vi "Periodic Tasks.vi"(8 "error in":errorcluster) -> ()   [LabVIEW 2016]
doc: "This VI runs in parallel to other tasks. It can contain as many user-defined periodic loops as you need. These can carry out PID or other sorts of timed response."
uses:
  <vilib>/Rock Robotics/WPI/AnalogOutput/WPI_AnalogOutputChannel.ctl
  <vilib>/Platform/TimedLoop/XDataNode/timing_clust.ctl
  <vilib>/Platform/TimedLoop/XDataNode/nitl_modes.ctl
  <vilib>/Platform/TimedLoop/XDataNode/wakeup.ctl
  <vilib>/Waveform/WDTFileIO.llb/Read Waveform from File.vi
  Robot Global Data.vi
  <vilib>/platform/TimedLoop/XDataNode/XDataNode.xnode
  <vilib>/Platform/TimedLoop/XDataNode/XDNodeRunTimeDep.lvlib
panel:
  in  "Volume":dbl(slide)=3.5 scale=0.0..3.0
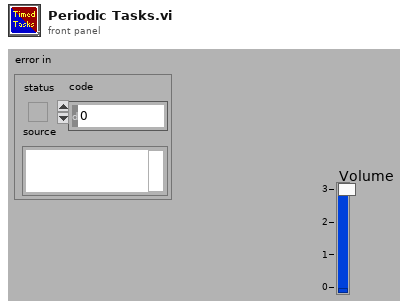
[diagram p1: front panel]
types:
  T1 = typedef "WPI_AnalogOutputChannel.ctl" = enum8{"AO MXP 0", "AO MXP 1", "Invalid"}
  T2 = typedef "JoystickData.ctl" = cluster{"X":dbl, "Y":dbl, "Z":dbl, "RestartMusic":bool}
  T3 = typedef "XDNodeRunTimeDep.lvlib/timing_clust.ctl" = cluster{"Expected End [f-1]":u64, "Actual End [f-1]":u64, "Finished Late? [f-1]":bool, "Expected End [i-1]":u64, "Actual End [i-1]":u64, "Finished Late? [i-1]":bool, "Expected Start [i]":u64, "Actual Start [i]":u64, "Expected Start [f]":u64, "Actual Start [f]":u64, "Source Name":string, "Structure Name":string, "Period":i64, "Deadline":i64, "Offset":i64, "Start":i64, "Priority":i32, "Timeout":i32, "Mode":T4, "Wakeup Reason":T5, "Error":errorcluster, "Source Type":string, "Secondary Source Type":string, "Global End Time":u64, "Global Start Time":u64, "Frame Duration":u64, "Iteration Duration":u64, "Assigned CPU":i32, "I/O Scan Engine Mode":u32}
  T4 = typedef "XDNodeRunTimeDep.lvlib/nitl_modes.ctl" = enum32{"No Change", "Process missed periods, maintain original phase", "Discard missed periods, maintain original phase", "Process missed periods, ignore original phase", "Discard missed periods, ignore original phase"}
  T5 = typedef "XDNodeRunTimeDep.lvlib/wakeup.ctl" = enum32{"Normal", "Aborted", "Asynchronous wakeup", "Timing source error", "Timed loop error", "Timeout"}
  T6 = typedef "WPI_AOChannelDevRef.ctl" = cluster{"DevStatus":errorcluster, "AO Channel":T1}
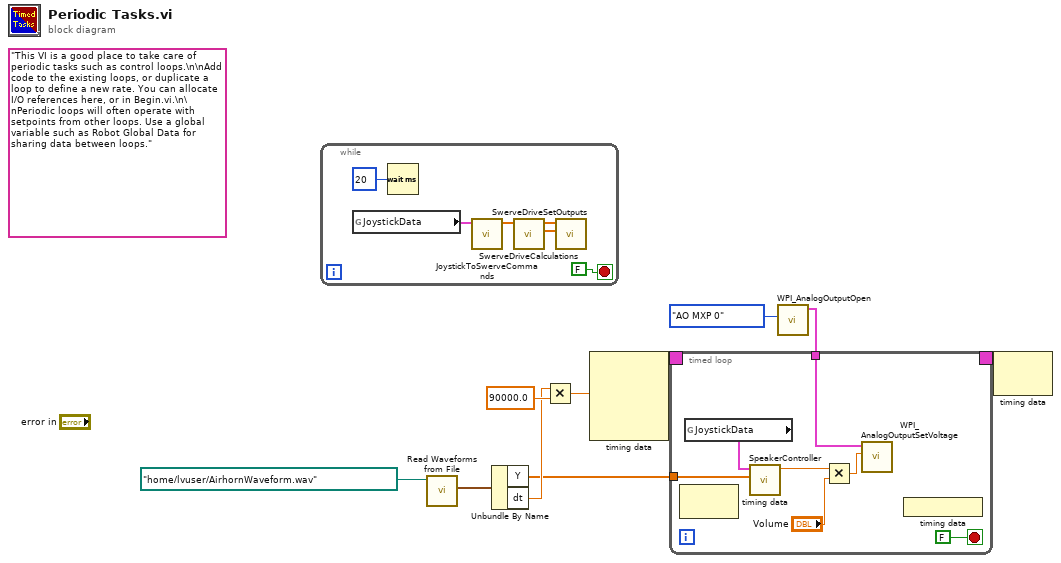
[diagram p0: block diagram]
diagram:
  (unwired) "This VI is a good place to take care of periodic tasks such as control loops.\n\nAdd code to the existing loops, or duplicate a loop to define a new rate. You can allocate I/O references here, or in Begin.vi.\n\nPeriodic loops will often operate with setpoints from other loops. Use a global variable such as Robot Global Data for sharing data between loops."
  n1 = while {
    stop <- FALSE stop-if-true
    n2 = global read "Robot Global Data.vi" "JoystickData"() -> (w14:T2)
    n3 = Wait (ms)(milliseconds to wait=u32 20) -> ()  [unwired: 1 out]
    n4 = call "JoystickToSwerveCommands.vi"("JoystickData"=w14) -> ("SwerveCommands"=w13:dbl[])  [unwired: 10 in]
    n5 = call "SwerveDriveCalculations.vi"("SwerveCommands"=w13) -> ("VelocitySetpoints"=w11:dbl[], "AngleSetpoints"=w12:dbl[])  [unwired: 9 in]
    n6 = call "SwerveDriveSetOutputs.vi"("VelocitySetpoints"=w11, "AngleSetpoints"=w12) -> ()  [unwired: 10 in]
  }
  n7 = call-poly <vilib>:"Read Waveforms from File.vi"("file path (dialog if empty)"=path "/home/lvuser/AirhornWaveform.wav") -> ("first waveform in record"=w3:waveform(dbl))  [unwired: 5 in, 3 out]
  n8 = Unbundle By Name(w3) -> ("Y"=w2:dbl[], "dt"=w7:dbl)
  n9 = Multiply(x=w7, y=90000.0) -> (x*y=w4:dbl)
  n10 = node-c288(w4) -> (w6:T3)  [unwired: 3 in]
  n11 = call <vilib>:"WPI_AnalogOutputOpen.vi"("AO Channel"=WPI_AnalogOutputChannel."AO MXP 0") -> ("AODeviceRef"=w1:T6)  [unwired: 9 in, 1 out]
  n12 = timed-loop {
    timing: w6 -> [_]
    timing-out: [_] -> w5
    tunnel: w2 -> [w20]
    tunnel: w1 -> [w19]
    stop <- FALSE stop-if-true
    n13 = node-c288() -> ()  [unwired: 1 in, 1 out]
    n14 = global read "Robot Global Data.vi" "JoystickData"() -> (w17:T2)
    n15 = call "SpeakerController.vi"("SongWaveform"=w20, "JoystickData"=w17) -> ("Voltage"=w21:dbl)  [unwired: 9 in]
    n16 = Multiply(x=w21, y="Volume") -> (x*y=w23:dbl)
    n17 = call <vilib>:"WPI_AnalogOutputSetVoltage.vi"("Voltage"=w23, "AODeviceRef"=w19) -> ()  [unwired: 8 in, 2 out]
    n18 = node-c288() -> ()  [unwired: 1 out]
  }
  n19 = node-c288(w5) -> ()  [unwired: 1 out]
